vi "Destroy.vi"(8 "error in":errorcluster, 11 "_Rescript Msg in":refnum<class "_Rescript Msg.lvclass">) -> (0 "error out":errorcluster)   [LabVIEW 2021, in "_Rescript Msg.lvlib" / "_Rescript Msg.lvclass"]
uses:
  _Rescript Msg.lvclass
  _Rescript Msg.lvclass/_Rescript Msg.ctl
  <vilib>/Utility/EditLVProj/Edit LVProj.lvlib
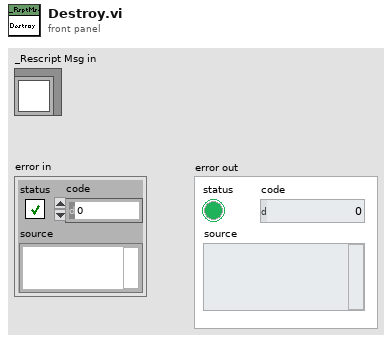
[diagram p1: front panel]
types:
  T1 = typedef "Edit LVProj.lvlib/Library And VI References.ctl" = cluster{"Target Reference":refnum<vi>, "VI References":refnum<vi>[], "Library References":refnum<vi>[]}
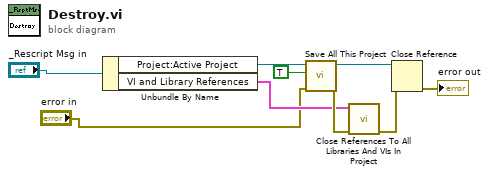
[diagram p0: block diagram]
diagram:
  n1 = Unbundle By Name("_Rescript Msg in") -> ("Project:Active Project"=w6:refnum<vi>, "VI and Library References"=w3:T1[])
  n2 = call <vilib>:"Save All This Project.vi"("error in (no error)"="error in", "Exclude Dependencies? (F)"=TRUE, "Project in"=w6) -> ("error out"=w8:errorcluster, "Project out"=w7:refnum<vi>)  [unwired: 7 in]
  n3 = call <vilib>:"Close References To All Libraries And VIs In Project.vi"("error in (no error)"=w8, "VI and Library References"=w3) -> ("error out"=w9:errorcluster)  [unwired: 9 in]
  n4 = Close Reference(reference=w7, error in (no error)=w9) -> (error out=→"error out":errorcluster)
